vi "SubVI_ProcessData.vi"(11 "Data Array":dbl[][](array[numeric])) -> (0 "dt":dbl, 1 "end time stamp":timestamp, 2 "start time stamp":timestamp, 3 "Data Array out":dbl[][](array[numeric]))   [LabVIEW 2012]
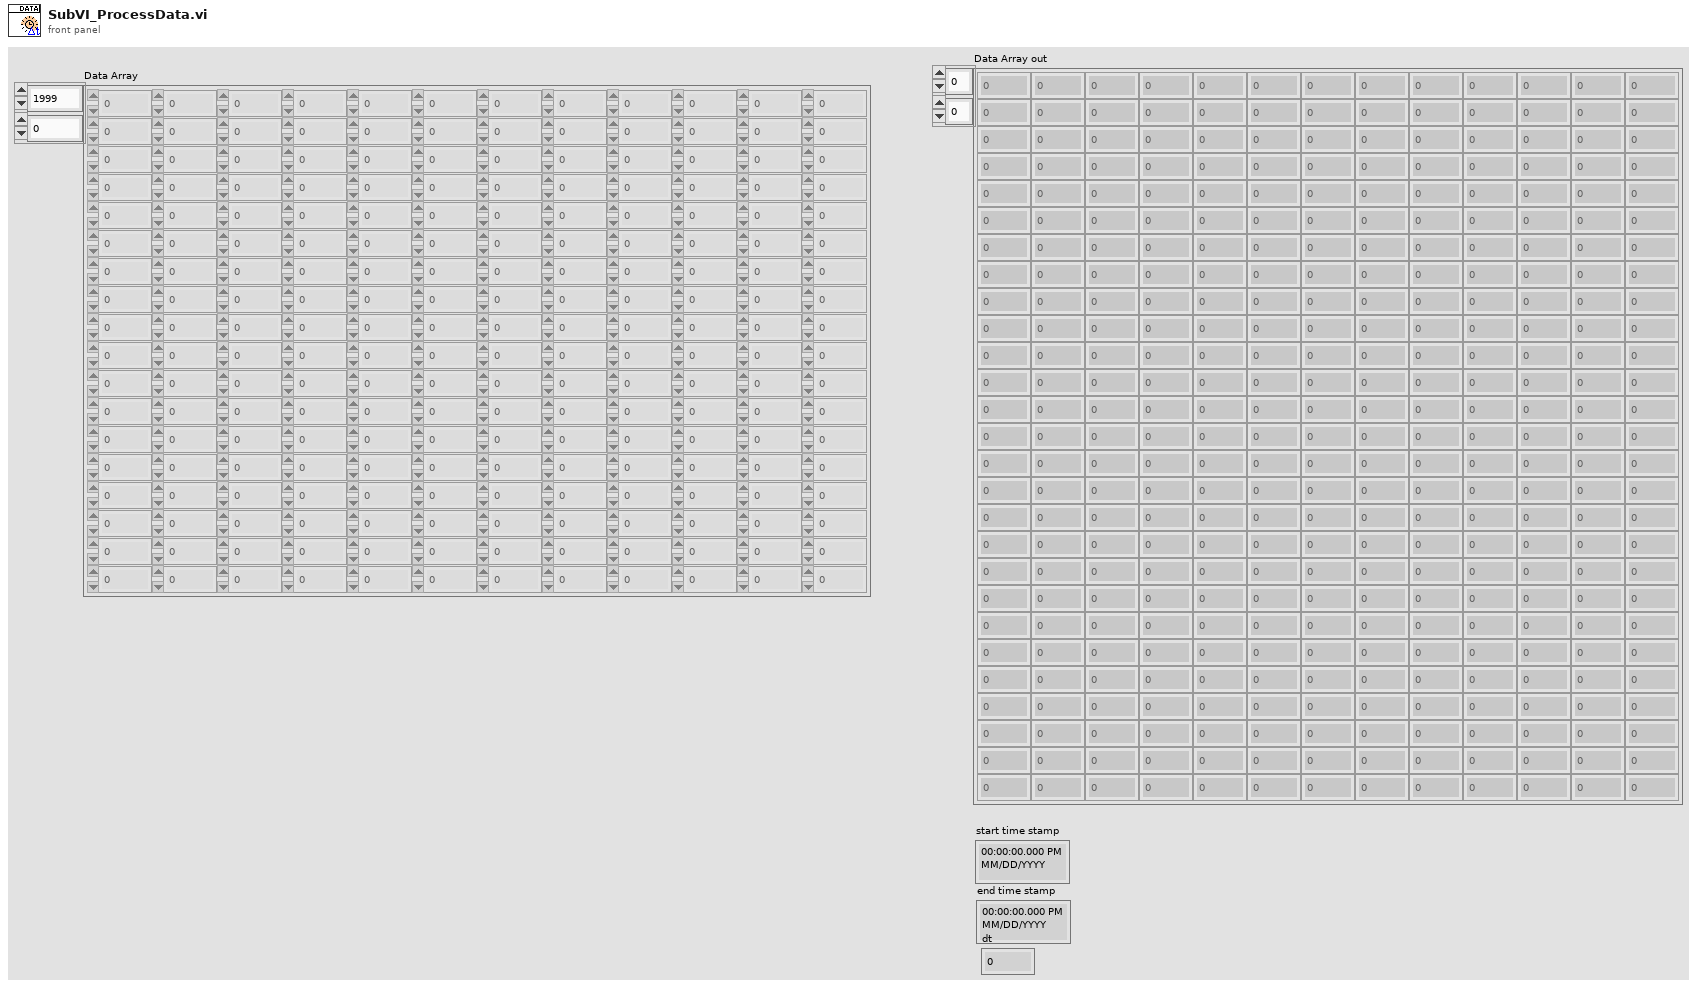
[diagram p1: front panel]
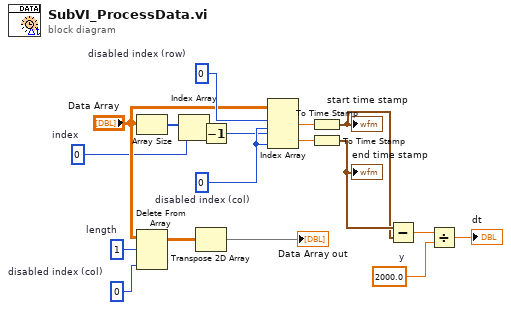
[diagram p0: block diagram]
diagram:
  w6 = 2000.0  # y
  w8 = 0  # index
  w14 = 0  # disabled index (row)
  w15 = 0  # disabled index (col)
  w17 = 0  # disabled index (col)
  w18 = 1  # length
  n1 = Array Size(array="Data Array") -> (size(s)=w12:i32[])
  n2 = Delete From Array(array="Data Array", length=w18, index (col)=w17) -> (array with subset deleted=w16:dbl[][])  [unwired: 1 in, 1 out]
  n3 = Index Array(array=w12, index=w8) -> (element=w11:i32)
  n4 = Transpose 2D Array(2D array=w16) -> (transposed array=→"Data Array out":dbl[][])
  n5 = Decrement(x=w11) -> (x-1=w1:i32)
  n6 = Index Array(array="Data Array", index (row) #1=w14, index (col) #1=w15, index (row) #2=w1, index (col) #2=w15) -> (element #1=w10:dbl, element #2=w9:dbl)
  n7 = To Time Stamp(1:w10) -> (0:w3:timestamp)
  "start time stamp" <- w3
  n8 = To Time Stamp(1:w9) -> (0:w4:timestamp)
  "end time stamp" <- w4
  n9 = Subtract(x=w4, y=w3) -> (x-y=w5:dbl)
  n10 = Divide(x=w5, y=w6) -> (x/y=→"dt":dbl)
